vi "Initialise Game Objects.vi"(8 "error in (no error)":errorcluster, 11 "Main Controller Actor in":refnum<class "Main Controller Actor.lvclass">) -> (0 "error out":errorcluster, 3 "Main Controller Actor out":refnum<class "Main Controller Actor.lvclass">)   [LabVIEW 2021, in "Main Controller Actor.lvclass"]
uses:
  Main Controller Actor.lvclass
  Main Controller Actor.lvclass/Main Controller Actor.ctl
  Ship/Ship.lvclass
  Asteroid/Asteroid.lvclass
  Planet/Planet.lvclass
  Renderer/Renderer.lvclass
  Element/Element.lvclass
  Element/Player Type.ctl
  Globals.vi
  Galaxy/Galaxy.lvclass
  Ship.ctl
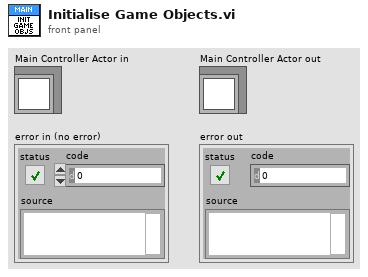
[diagram p1: front panel]
types:
  T1 = typedef "Main Controller Actor.lvclass/Ship.ctl" = enum16{"Arilou", "Chmmr", "Kohrah", "Slylandro"}
  T2 = typedef "Element.lvclass/Player Type.ctl" = enum16{"Neutral", "Player 1", "Player 2"}
  T3 = typedef "Constants.ctl" = cluster{"Colours":cluster{"OK":u32, "Warning":u32, "Error":u32, "Red":u32, "Green":u32, "Blue":u32, "Yellow":u32}, "System":cluster{"Target Frames Second":dbl, "World Size":T4, "Window Size":T4, "Battle Area Size":T4, "Sidebar Scaling":sgl, "Sidebar Width":i32, "SC2 Frame Rate [Seconds/Frame]":sgl}, "Game":cluster{"Maximum Asteroids":i32, "Max Energy":i32, "Max Crew":i32, "Maximum Stars":i32}}
  T4 = typedef "SDL2 Utility.lvlib/Point (I32).ctl" = cluster{"x":i32, "y":i32}
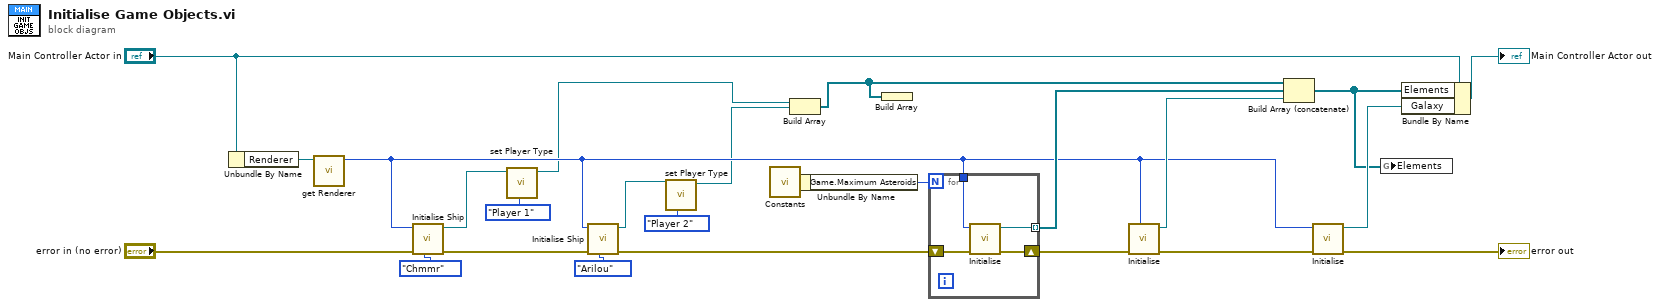
[diagram p0: block diagram]
diagram:
  n1 = Unbundle By Name("Main Controller Actor in") -> ("Renderer"=w23:refnum<class "Renderer.lvclass">)
  n2 = call-dynamic "get Renderer.vi"("Renderer in"=w23) -> ("Renderer"=w8:u32)  [unwired: 10 in]
  n3 = call "Initialise Ship.vi"("Ship"=Ship."Chmmr", "error in (no error)"="error in (no error)", "Renderer"=w8) -> ("error out"=w12:errorcluster, "Ship"=w10:refnum<class "Ship.lvclass">)  [unwired: 7 in]
  n4 = call "set Player Type.vi"("Player Type"=Player_Type."Player 1", "Element in"=w10) -> ("Element out"=w3:refnum<class "Ship.lvclass">)  [unwired: 9 in]
  n5 = call "Initialise Ship.vi"("Ship"=Ship."Arilou", "error in (no error)"=w12, "Renderer"=w8) -> ("error out"=w11:errorcluster, "Ship"=w9:refnum<class "Ship.lvclass">)  [unwired: 7 in]
  n6 = call "set Player Type.vi"("Player Type"=Player_Type."Player 2", "Element in"=w9) -> ("Element out"=w7:refnum<class "Ship.lvclass">)  [unwired: 9 in]
  n7 = call "Constants.vi"() -> ("Constants"=w5:T3)
  n8 = Build Array(w3, w7) -> (w2:refnum<class "Ship.lvclass">[])
  n9 = Unbundle By Name(w5) -> ("Game.Maximum Asteroids"=w4:i32)
  n10 = Build Array(w2) -> ()  [unwired: 1 out]
  n11 = for {
    N: w4 -> [_]
    shift-right: [w29] -> w25
    shift-left: w11 -> [w28]
    tunnel: [w27] -> w22 mode=indexing
    tunnel: w8 -> [w26]
    n12 = call "Initialise.vi"("error in (no error)"=w28, "Renderer"=w26) -> ("error out"=w29:errorcluster, "Asteroid out"=w27:refnum<class "Asteroid.lvclass">)  [unwired: 8 in]
  }
  n13 = call "Initialise.vi"("Renderer"=w8, "error in (no error)"=w25) -> ("error out"=w20:errorcluster, "Planet out"=w21:refnum<class "Planet.lvclass">)  [unwired: 8 in]
  n14 = Build Array (concatenate)(w2, w22, w21) -> (w1:refnum<class "Element.lvclass">[])
  n15 = call "Initialise.vi"("error in (no error)"=w20, "Renderer"=w8) -> ("error out"=→"error out":errorcluster, "Galaxy out"=w18:refnum<class "Galaxy.lvclass">)  [unwired: 8 in]
  n16 = global write "Globals.vi" "Elements"(w1) -> ()
  n17 = Bundle By Name(cluster="Main Controller Actor in", "Elements"=w1, "Galaxy"=w18) -> (→"Main Controller Actor out":refnum<class "Main Controller Actor.lvclass">)
